vi "add_name_explistSD.vi"(3 "Exp name":string, 4 "exp #":i32, 5 "Item Names in":string[](array[string])) -> (0 "Item Names out":string[](array[string]), 1 "name out":string, 2 "Numeric":i32)   [LabVIEW 2015]
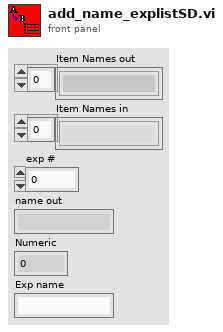
[diagram p1: front panel]
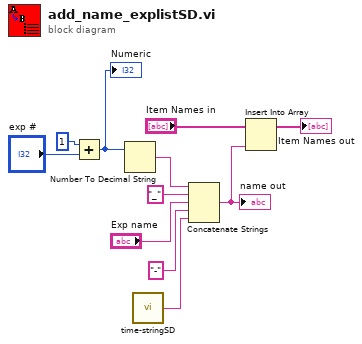
[diagram p0: block diagram]
diagram:
  n1 = Add(x=1, y="exp #") -> (x+y=w10:i32)
  "Numeric" <- w10
  n2 = Number To Decimal String(number=w10) -> (decimal integer string=w4:string)  [unwired: 1 in]
  n3 = call "time-stringSD.vi"() -> ("time"=w7:string)
  n4 = Concatenate Strings(w4, "_" ("string"), "Exp name", "-" ("string"), w7) -> (w2:string)
  "name out" <- w2
  n5 = Insert Into Array(array="Item Names in", new element=w2) -> (→"Item Names out":string[])  [unwired: 1 in]
